vi "Untitled 6 (SubVI).vi"(8 "error in (no error)":errorcluster, 10 "Boolean":bool, 11 "VI in":refnum<vi>) -> (0 "error out":errorcluster, 3 "VI in 2":refnum<vi>)   [LabVIEW 2015]
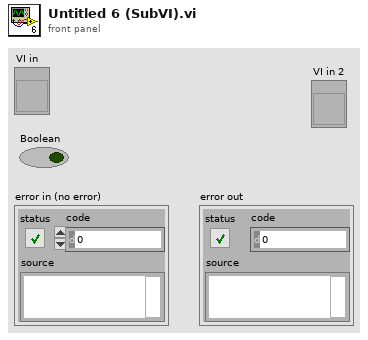
[diagram p1: front panel]
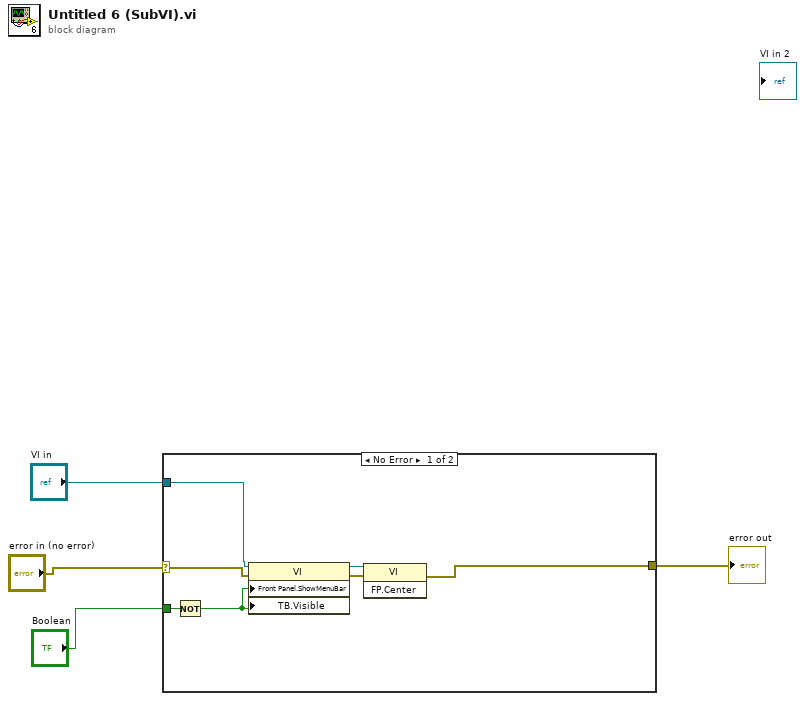
[diagram p0: block diagram]
diagram:
  n1 = case shown="No Error" "error in (no error)" {
    selector: "error in (no error)" -> [w6 w12]
    tunnel: [w10 w12] -> w4
    tunnel: "VI in" -> [w9 _]
    tunnel: "Boolean" -> [w7 _]
    frame No Error {
      n2 = Not(x=w7) -> (.not. x?=w5:bool)
      n3 = property class="VI"(reference=w9, error in=w6, "Front Panel.ShowMenuBar"=w5, "TB.Visible"=w5) -> (reference out=w11:refnum<vi>, error out=w8:errorcluster)
      n4 = invoke class="VI" method="FP.Center"(reference=w11, error in=w8) -> (error out=w10:errorcluster)  [unwired: 1 in, 2 out]
    }
    frame Error {
    }
  }
  "error out" <- w4
